vi "music.NoteOff.vi"(8 "error in (no error)":errorcluster, 10 "key":i32, 11 "midi-ui in":refnum<class "midi-ui.lvclass">) -> (0 "error out":errorcluster, 3 "midi-ui out":refnum<class "midi-ui.lvclass">)   [LabVIEW 2020, in "midi-ui.lvclass"]
uses:
  midi-ui.lvclass
  midi-ui.lvclass/midi-ui.ctl
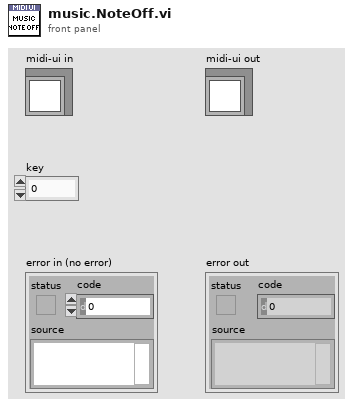
[diagram p1: front panel]
types:
  T1 = map{i32, cluster{"Note On":picture, "Note Off":picture}}
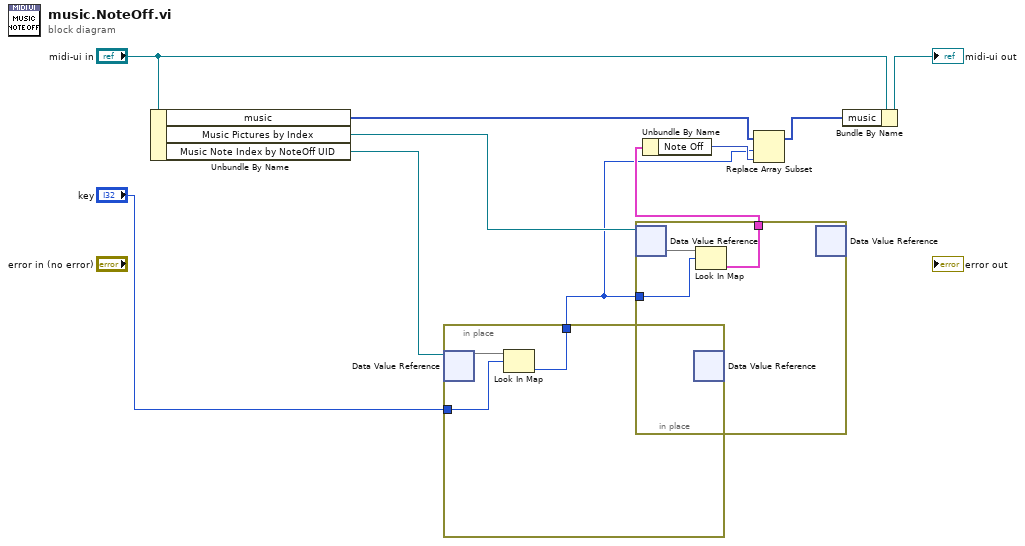
[diagram p0: block diagram]
diagram:
  n1 = Unbundle By Name("midi-ui in") -> ("music"=w4:picture[], "Music Pictures by Index"=w8:refnum<data-value>, "Music Note Index by NoteOff UID"=w7:refnum<data-value>)
  n2 = in-place {
    in-place-border: [w13] -> w2
    in-place-border: "key" -> [w11]
    n3 = in-place-dvr #1(w7) -> (w12:map{i32, i32})  [unwired: 1 out]
    n4 = Look In Map(map=w12, key=w11) -> (value=w13:i32)  [unwired: 1 in, 1 out]
    n5 = in-place-dvr #1() -> ()  [unwired: 1 in, 2 out]
  }
  n6 = in-place {
    in-place-border: [w16] -> w5
    in-place-border: w2 -> [w14]
    n7 = in-place-dvr #2(w8) -> (w15:T1)  [unwired: 1 out]
    n8 = Look In Map(map=w15, key=w14) -> (value=w16:cluster{"Note On":picture, "Note Off":picture})  [unwired: 1 in, 1 out]
    n9 = in-place-dvr #2() -> ()  [unwired: 1 in, 2 out]
  }
  n10 = Unbundle By Name(w5) -> ("Note Off"=w3:picture)
  n11 = Replace Array Subset(array=w4, new element=w3, index=w2) -> (w1:picture[])
  n12 = Bundle By Name(cluster="midi-ui in", "music"=w1) -> (→"midi-ui out":refnum<class "midi-ui.lvclass">)
